vi "Module Did Stop.vi"(8 "error in (no error)":errorcluster, 10 "Origin":string) -> (0 "error out":errorcluster)   [LabVIEW 2020, in "Paquetes Disponibles.lvlib"]
doc: "Send the Module Did Stop event to any VI registered to listen to this module's broadcast events.\n_____\nBased on DQMH Project Template 6.0.0.91."
uses:
  Paquetes Disponibles.lvlib
  Stop Argument--cluster.ctl
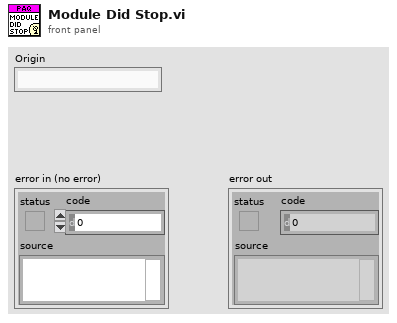
[diagram p1: front panel]
types:
  T1 = typedef "Paquetes Disponibles.lvlib/Stop Argument--cluster.ctl" = cluster{"Origin":string, "Exit via Stop Module Req?":bool, "Wait for Module to stop?":bool}
  T2 = typedef "Paquetes Disponibles.lvlib/Broadcast Events--cluster.ctl" = cluster{"Module Did Init":refnum<user-event>, "Status Updated":refnum<user-event>, "Error Reported":refnum<user-event>, "Module Did Stop":refnum<user-event>, "Update Module Execution Status":refnum<user-event>, "Servicio Seleccionado":refnum<user-event>, "Actualizar Credito":refnum<user-event>, "Actualizar Cambio":refnum<user-event>}
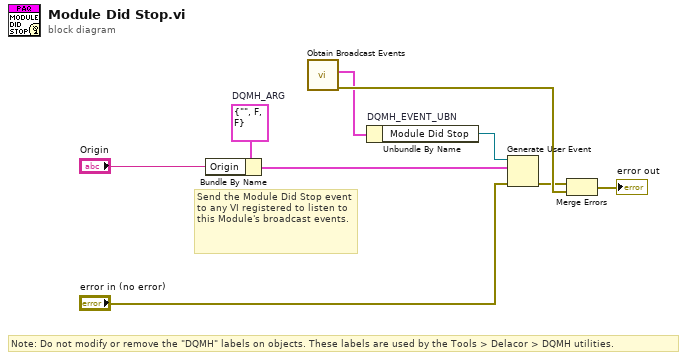
[diagram p0: block diagram]
diagram:
  w2 = T1 {"Origin"="", "Exit via Stop Module Req?"=FALSE, "Wait for Module to stop?"=FALSE}  # DQMH_ARG
  # "Note: Do not modify or remove the \"DQMH\" labels on objects. These labels are used by the Tools > Delacor > DQMH utilities."
  # "Send the Module Did Stop event to any VI registered to listen to this Module's broadcast events."
  n1 = Bundle By Name(cluster=w2, "Origin"="Origin") -> (w3:T1)
  n2 = call "Obtain Broadcast Events.vi"() -> ("error out"=w9:errorcluster, "Paquetes Disponibles Broadcast Events"=w5:T2)  [unwired: 10 in]
  n3 = Unbundle By Name "DQMH_EVENT_UBN"(w5) -> ("Module Did Stop"=w4:refnum<user-event>)
  n4 = Generate User Event(user event=w4, event data cluster=w3, error in="error in (no error)") -> (error out=w6:errorcluster)  [unwired: 1 in, 1 out]
  n5 = Merge Errors(w6, w9) -> (→"error out":errorcluster)
